vi "ControlMotorPivot.vi"(11 "POVs23":i16[](array[numeric])) -> ()   [LabVIEW 2015]
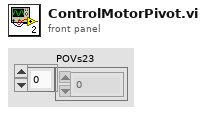
[diagram p1: front panel]
types:
  T1 = typedef "WPI_MotorControlDeviceRef.ctl" = cluster{"DeviceStatus":errorcluster, "Type":T2, "PWM":cluster{"PWM Channel":T3, "DeadBand":T4}, "CAN":cluster{"Device Number":u8, "Control Mode":T5, "Semaphore":T6, "Max Vout":dbl, "TalonSRX Control Mode":T7}, "Invert":bool}
  T2 = typedef "WPI_MotorControlType.ctl" = enum16{"PWM", "CAN", "CANTalonSRX"}
  T3 = typedef "FPGA_DIOPWMChannel.ctl" = enum8{"PWM 0", "PWM 1", "PWM 2", "PWM 3", "PWM 4", "PWM 5", "PWM 6", "PWM 7", "PWM 8", "PWM 9", "PWM MXP 0", "PWM MXP 1", "PWM MXP 2", "PWM MXP 3", "PWM MXP 4", "PWM MXP 5", "PWM MXP 6", "PWM MXP 7", "PWM MXP 8", "PWM MXP 9", "Invalid"}
  T4 = typedef "WPI_PWMDeadband.ctl" = cluster{"Name":string, "maxPositivePwm":i32, "minPositivePwm":i32, "centerPwm":i32, "maxNegativePwm":i32, "minNegativePwm":i32, "angularRange":u16}
  T5 = typedef "WPI_CANJaguar_ControlMode.ctl" = enum8{"Percent VBus", "Current", "Speed", "Position", "Voltage"}
  T6 = typedef "Semaphore RefNum" = refnum<k1>
  T7 = typedef "WPI_CANTalonSRX_APIControlMode.ctl" = enum8{"Percent VBus", "Speed", "Position", "Slave", "Unchanged / Invalid", "Voltage Compensation", "Current", "Motion Profile"}
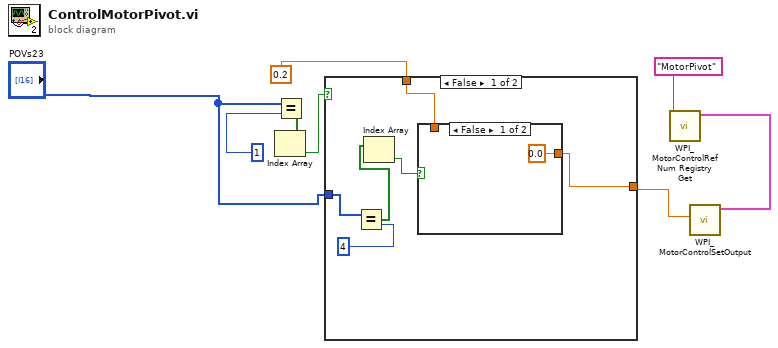
[diagram p0: block diagram]
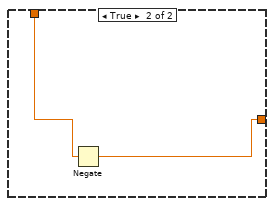
[diagram p3: hidden frame]
diagram:
  n1 = Equal?(x="POVs23", y=1) -> (x = y?=w1:bool[])
  n2 = Index Array(array=w1) -> (element=w2:bool)  [unwired: 1 in]
  n3 = case shown="False" w2 {
    tunnel: "POVs23" -> [w13 _]
    tunnel: 0.2 -> [w10 w18]
    tunnel: [w9 w17] -> w7
    frame False {
      n4 = Equal?(x=w13, y=4) -> (x = y?=w12:bool[])
      n5 = Index Array(array=w12) -> (element=w11:bool)  [unwired: 1 in]
      n6 = case shown="False" w11 {
        tunnel: [0.0 w16] -> w9
        tunnel: w10 -> [_ w16]
        frame False {
        }
        frame True {
        }
      }
    }
    frame True {
      n7 = Negate(x=w18) -> (-x=w17:dbl)
    }
  }
  n8 = call <vilib>:"WPI_MotorControlRefNum Registry Get.vi"("refnum name"="MotorPivot") -> ("MotorControlDevRef"=w8:T1)  [unwired: 9 in, 1 out]
  n9 = call <vilib>:"WPI_MotorControlSetOutput.vi"("Output"=w7, "MotorControlDevRef"=w8) -> ()  [unwired: 7 in, 3 out]
